vi "SPITest.vi"() -> ()   [LabVIEW 2013]
uses:
  <vilib>/Rock Robotics/SystemInterfaces/DIO/FPGA_DIOChannel.ctl
  <vilib>/Rock Robotics/WPI/SPI/WPI_SPIBits Per Word.ctl
panel:
  out "error out 2":errorcluster
  out "Received Data":u32
  out "error out":errorcluster
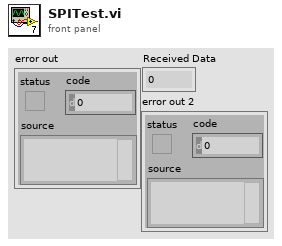
[diagram p1: front panel]
types:
  T1 = typedef "WPI_SPIBits Per Word.ctl" = u8
  T2 = typedef "FPGA_DIOChannel.ctl" = enum8{"DIO 1", "DIO 2", "DIO 3", "DIO 4", "DIO 5", "DIO 6", "DIO 7", "DIO 8", "DIO 9", "DIO 10", "DIO 11", "DIO 12", "DIO 13", "DIO 14", "Invalid"}
  T3 = typedef "WPI_DigitalInputDevRef.ctl" = cluster{"DevStatus":errorcluster, "DIO Channel":T2, "Digital Module":T4}
  T4 = typedef "FPGA_TypedefDigitalModule.ctl" = enum16{"Digital Module 1", "Digital Module 2"}
  T5 = typedef "WPI_DigitalOutputDevRef.ctl" = cluster{"Digital Module":T4, "DIO Channel":T2, "DevStatus":errorcluster}
  T6 = typedef "WPI_SPIDevRef.ctl" = cluster{"DevStatus":errorcluster}
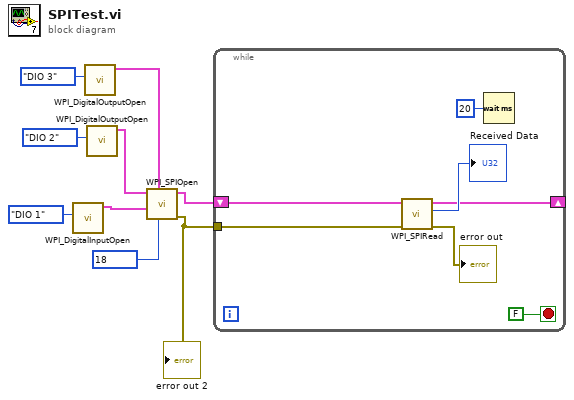
[diagram p0: block diagram]
diagram:
  w3 = T1 18 items=["8-Bit"=8, "16-Bit"=16, "32-Bit"=32] ("Bits Per Word")
  n1 = call <vilib>:"WPI_DigitalInputOpen.vi"("DIO Channel"=FPGA_DIOChannel."DIO 1") -> ("DigitalInputDevRef"=w4:T3)  [unwired: 9 in, 1 out]
  n2 = call <vilib>:"WPI_DigitalOutputOpen.vi"("DIO Channel"=FPGA_DIOChannel."DIO 3") -> ("DigitalOutputDevRef"=w8:T5)  [unwired: 9 in, 1 out]
  n3 = call <vilib>:"WPI_DigitalOutputOpen.vi"("DIO Channel"=FPGA_DIOChannel."DIO 2") -> ("DigitalOutputDevRef"=w6:T5)  [unwired: 9 in, 1 out]
  n4 = call <vilib>:"WPI_SPIOpen.vi"("Bits Per Word"=w3, "Chip Select"=w8, "Master-In Slave-Out"=w4, "Clock"=w6) -> ("error out"=w1:errorcluster, "SPIDevRef"=w2:T6)  [unwired: 6 in]
  "error out 2" <- w1
  n5 = while {
    tunnel: w1 -> [w13]
    shift-right: [w10] -> _
    shift-left: w2 -> [w14]
    stop <- FALSE stop-if-true
    n6 = call <vilib>:"WPI_SPIRead.vi"("error in (no error)"=w13, "SPIDevRef"=w14) -> ("error out"=→"error out":errorcluster, "Received Data"=→"Received Data":u32, "SPIDevRef"=w10:T6)  [unwired: 7 in]
    n7 = Wait (ms)(milliseconds to wait=u32 20) -> ()  [unwired: 1 out]
  }
